vi "getShape.vi"(8 "error in (no error)":errorcluster, 10 "Shape":string, 11 "ColorFactory in":refnum<class "ColorFactory.lvclass">) -> (0 "error out":errorcluster, 2 "afShape.lvclass":refnum<class "afShape.lvclass">, 3 "ColorFactory out":refnum<class "ColorFactory.lvclass">)   [LabVIEW 2018, in "ColorFactory.lvclass"]
uses:
  ColorFactory.lvclass
  afShape Class/afShape.lvclass
  AbstractFactory Class/AbstractFactory.lvclass
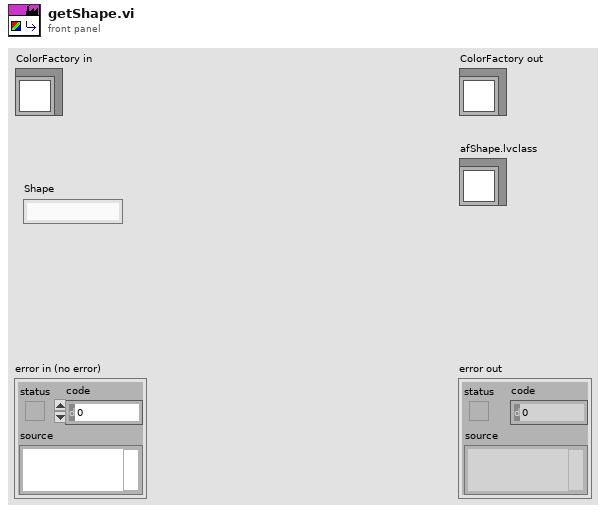
[diagram p1: front panel]
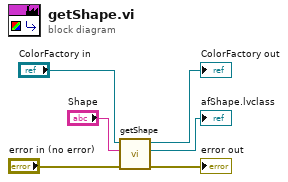
[diagram p0: block diagram]
diagram:
  n1 = call-parent "getShape.vi"("error in (no error)"="error in (no error)", "Shape"="Shape", "AbstractFactory in"="ColorFactory in") -> ("error out"=→"error out":errorcluster, "afShape.lvclass"=→"afShape.lvclass":refnum<class "afShape.lvclass">, "AbstractFactory out"=→"ColorFactory out":refnum<class "ColorFactory.lvclass">)  [unwired: 6 in]
